vi "circularMemoryCounter.vi"(7 "reset":bool, 8 "doStep":bool=TRUE, 9 "foward":bool=TRUE, 10 "start":u16, 11 "maxCount":u16) -> (0 "maxReached":bool, 2 "next":u16, 3 "index":u16)   [LabVIEW 2016]
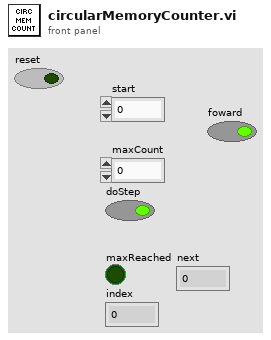
[diagram p1: front panel]
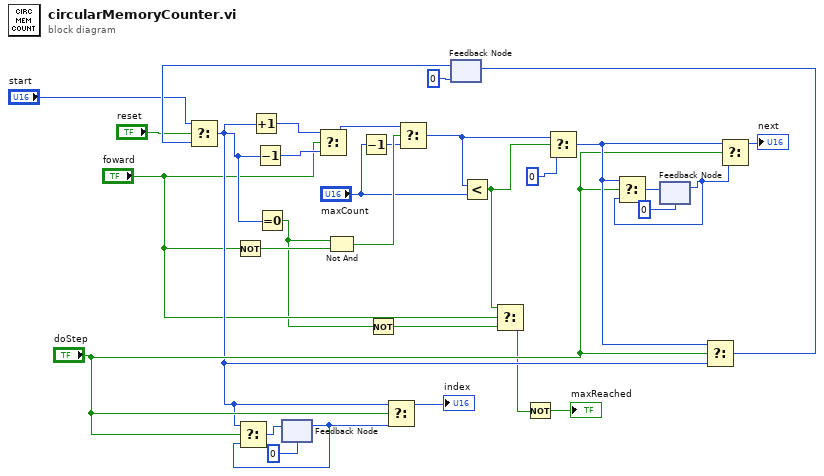
[diagram p0: block diagram]
diagram:
  n1 = Not(x="foward") -> (.not. x?=w10:bool)
  n2 = feedback #1(u16 0 ("t")) -> (w21:u16)
  n3 = Decrement(x="maxCount") -> (x-1=w6:u16)
  n4 = feedback #2(u16 0) -> (w29:u16)
  n5 = Select(t="start", s="reset", f=w29) -> (s? t:f=w11:u16)
  n6 = Select(t=w11, s="doStep", f=w21) -> (s? t:f=w22:u16)
  n7 = Increment(x=w11) -> (x+1=w30:u16)
  n8 = Decrement(x=w11) -> (x-1=w12:u16)
  n9 = Equal To 0?(x=w11) -> (x = 0?=w2:bool)
  n10 = feedback-in #1(w22) -> ()
  n11 = Select(t=w30, s="foward", f=w12) -> (s? t:f=w13:u16)
  n12 = Not And(1:w10, 2:w2) -> (0:w8:bool)
  n13 = Not(x=w2) -> (.not. x?=w1:bool)
  n14 = Select(t=w11, s="doStep", f=w21) -> (s? t:f=→"index":u16)
  n15 = Select(t=w13, s=w8, f=w6) -> (s? t:f=w9:u16)
  n16 = Less?(x=w9, y="maxCount") -> (x < y?=w4:bool)
  n17 = Select(t=w4, s="foward", f=w1) -> (s? t:f=w5:bool)
  n18 = Not(x=w5) -> (.not. x?=→"maxReached":bool)
  n19 = Select(t=w9, s=w4, f=u16 0) -> (s? t:f=w20:u16)
  n20 = feedback #3(u16 0) -> (w17:u16)
  n21 = Select(t=w20, s="doStep", f=w17) -> (s? t:f=w18:u16)
  n22 = feedback-in #3(w18) -> ()
  n23 = Select(t=w20, s="doStep", f=w11) -> (s? t:f=w27:u16)
  n24 = feedback-in #2(w27) -> ()
  n25 = Select(t=w20, s="doStep", f=w17) -> (s? t:f=→"next":u16)
